vi "Get TEMP path from ENV.vi"() -> (1 "TEMP Path":path)   [LabVIEW 2011]
uses:
  kernel32.dll
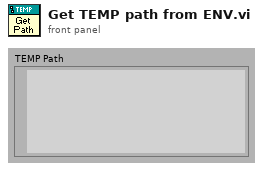
[diagram p1: front panel]
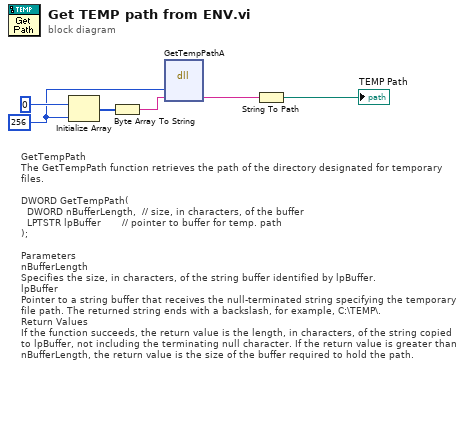
[diagram p0: block diagram]
diagram:
  w3 = u32 256 ("Dimension Size")
  # "GetTempPath\nThe GetTempPath function retrieves the path of the directory designated for temporary files. \n\nDWORD GetTempPath(\n  DWORD nBufferLength,  // size, in characters, of the buffer\n  LPTSTR lpBuffer       // pointer to buffer for temp. path\n);\n \nParameters\nnBufferLength \nSpecifies the size, in characters, of the string buffer identified by lpBuffer. \nlpBuffer \nPointer to a string buffer that receives the null-terminated string specifying the temporary file path. The returned string ends with a backslash, for example, C:\\TEMP\\. \nReturn Values\nIf the function succeeds, the return value is the length, in characters, of the string copied to lpBuffer, not including the terminating null character. If the return value is greater than nBufferLength, the return value is the size of the buffer required to hold the path."
  n1 = Initialize Array(u8 0, w3) -> (w4:u8[])
  n2 = Byte Array To String(unsigned byte array=w4) -> (string=w2:string)
  n3 = dll-call lib="kernel32.dll" fn="GetTempPathA"("nBufferLength"=w3, "lpBuffer"=w2) -> ("lpBuffer"=w6:string)  [unwired: 4 in, 3 out]
  n4 = String To Path(string=w6) -> (path=→"TEMP Path":path)
